vi "testRegisterCommand.vi"(8 "error in (no error)":errorcluster) -> (0 "error out":errorcluster)   [LabVIEW 2018]
doc: "Test the registerCommand.vi."
uses:
  src/TcpServer/TcpServer.lvclass
  src/TcpServer/TcpServer.lvclass/TcpServer.ctl
  <vilib>/addons/_JKI Toolkits/Caraya/classes/Assert/Assert Equal Value_Variant.vi
  <vilib>/addons/_JKI Toolkits/Caraya/classes/Test/Test.lvclass
  <vilib>/addons/_JKI Toolkits/Caraya/classes/Assert/Assert.lvclass
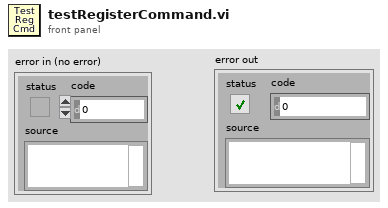
[diagram p1: front panel]
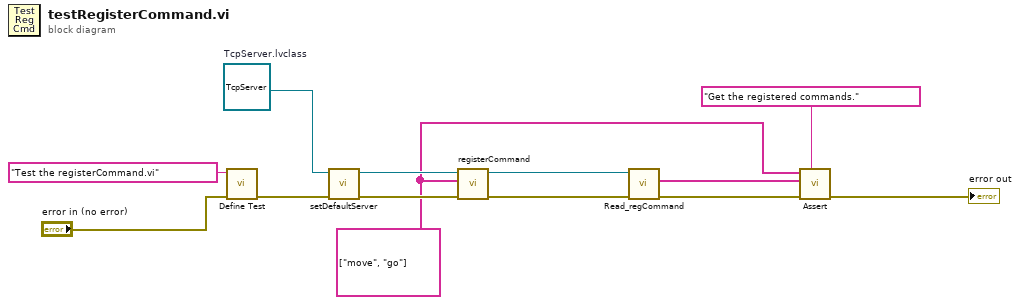
[diagram p0: block diagram]
diagram:
  w2 = string[] ["move", "go"] ("registeredCommands")
  w10 = refnum<class "TcpServer.lvclass"> refnum  # TcpServer.lvclass
  n1 = call <vilib>:"Define Test.vi"("error in (no error)"="error in (no error)", "Label (VI Title)"="Test the registerCommand.vi") -> ("error out"=w12:errorcluster)  [unwired: 9 in]
  n2 = call "setDefaultServer.vi"("error in (no error)"=w12, "TcpServer.lvclass"=w10) -> ("error out"=w7:errorcluster, "tcpServer out"=w8:refnum<class "TcpServer.lvclass">)  [unwired: 8 in]
  n3 = call "registerCommand.vi"("error in (no error)"=w7, "registeredCommands"=w2, "tcpServer in"=w8) -> ("error out"=w6:errorcluster, "tcpServer out"=w3:refnum<class "TcpServer.lvclass">)  [unwired: 7 in]
  n4 = call "Read_regCommand.vi"("error in (no error)"=w6, "TcpServer in"=w3) -> ("error out"=w4:errorcluster, "regCommand"=w1:string[])  [unwired: 7 in, 1 out]
  n5 = call-poly <vilib>:"Assert.vi"("Label"="Get the registered commands.", "error in (no error)"=w4, "Y"=w1, "X"=w2) -> ("error out"=→"error out":errorcluster)  [unwired: 7 in]
